vi "createMissionWaypoints.vi"(8 "error in (no error)":errorcluster, 11 "PassBuoys in":refnum<class "PassBuoys.lvclass">) -> (0 "error out":errorcluster, 3 "PassBuoys out":refnum<class "PassBuoys.lvclass">)   [LabVIEW 2011, in "PassBuoys.lvclass"]
doc: "Creates three waypoint objects for the mission, and puts them in the queue. The first waypoint is in front of the two buoys. The second is at their midpoint. The third is just past them."
uses:
  PassBuoys.lvclass
  PassBuoys.lvclass/PassBuoys.ctl
  2 Globals/2 Global.vi
  Waypoint/Waypoint.lvclass
panel:
  in  "Tolerance (meters)":dbl=3.0
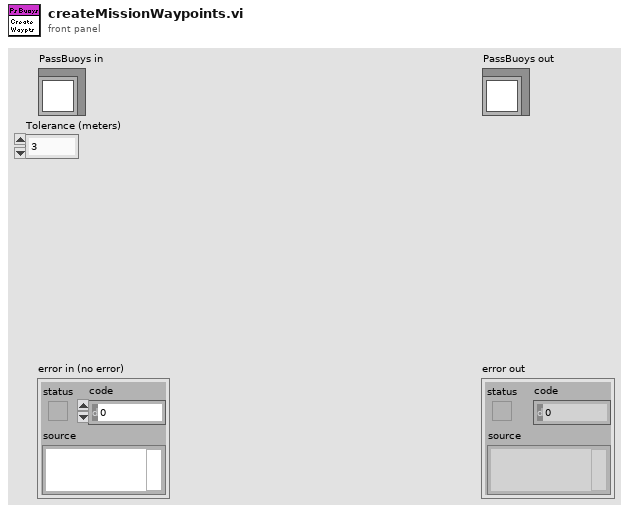
[diagram p1: front panel]
types:
  T1 = typedef "UTM Location.ctl" = cluster{"UTM Zone":dbl, "Hemisphere":enum16{"North", "South"}, "East":dbl, "North":dbl}
  T2 = typedef "UTM Circle.ctl" = cluster{"UTM Zone":dbl, "Hemisphere":enum16{"North", "South"}, "East":dbl, "North":dbl, "Radius":dbl}
  T3 = typedef "Waypoints List.ctl" = refnum<class "Waypoint.lvclass">[]
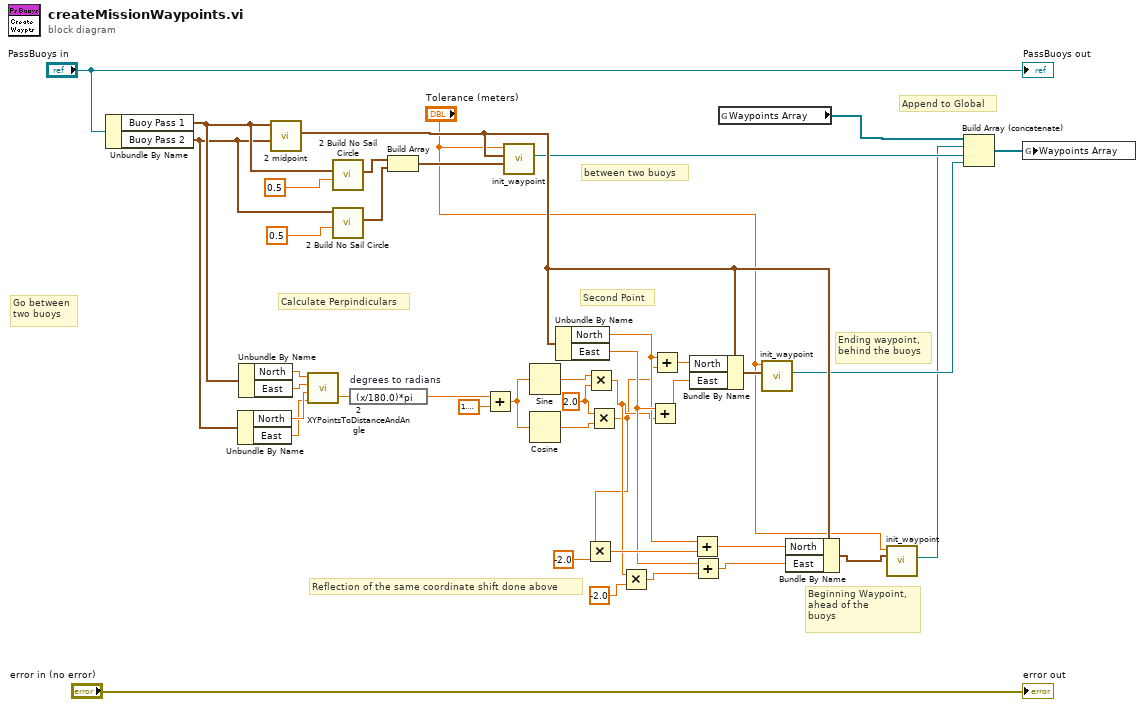
[diagram p0: block diagram]
diagram:
  w24 = 2.0 ("Tolerance (meters?)")
  # "Reflection of the same coordinate shift done above"
  # "between two buoys"
  # "Calculate Perpindiculars"
  # "Ending waypoint,\nbehind the buoys"
  # "Beginning Waypoint,\nahead of the\nbuoys"
  # "Second Point"
  # "Go between\ntwo buoys"
  # "Append to Global"
  n1 = Unbundle By Name("PassBuoys in") -> ("Buoy Pass 1"=w9:T1, "Buoy Pass 2"=w8:T1)
  n2 = Unbundle By Name(w8) -> ("North"=w32:dbl, "East"=w31:dbl)
  n3 = Unbundle By Name(w9) -> ("North"=w34:dbl, "East"=w33:dbl)
  n4 = call "2 midpoint.vi"("UTM 2"=w8, "UTM 1"=w9) -> ("Midpoint"=w15:T1)  [unwired: 8 in, 1 out]
  n5 = call "2 XYPointsToDistanceAndAngle.vi"("East 2"=w31, "North 2"=w32, "East 1"=w33, "North 1"=w34) -> ("Angle Diff"=w2:dbl)  [unwired: 1 out]
  n6 = call "2 Build No Sail Circle.vi"("Radius"=0.5, "UTM Location"=w9) -> ("UTM Circle"=w40:T2)  [unwired: 9 in]
  n7 = call "2 Build No Sail Circle.vi"("Radius"=0.5, "UTM Location"=w8) -> ("UTM Circle"=w38:T2)  [unwired: 9 in]
  n8 = expression code="(x/180.0)*pi" "degrees to radians"(w2) -> (w3:dbl)
  n9 = Build Array(w40, w38) -> (w41:T2[])
  n10 = Add(x=w3, y=1.5707963267948966) -> (x+y=w30:dbl)
  n11 = call "init_waypoint.vi"("No Sail Circles"=w41, "Coords"=w15, "Tolerance (m)"="Tolerance (meters)") -> ("Waypoint Out"=w12:refnum<class "Waypoint.lvclass">)  [unwired: 8 in]
  n12 = Sine(x=w30) -> (sin(x)=w26:dbl)
  n13 = Cosine(x=w30) -> (cos(x)=w25:dbl)
  n14 = Unbundle By Name(w15) -> ("North"=w18:dbl, "East"=w19:dbl)
  n15 = Multiply(x=w26, y=w24) -> (x*y=w6:dbl)
  n16 = Multiply(x=w24, y=w25) -> (x*y=w5:dbl)
  n17 = Multiply(x=w5, y=-2.0 ("Tolerance (meters?)")) -> (x*y=w20:dbl)
  n18 = Multiply(x=w6, y=-2.0 ("Tolerance (meters?)")) -> (x*y=w21:dbl)
  n19 = Add(x=w19, y=w6) -> (x+y=w29:dbl)
  n20 = Add(x=w18, y=w5) -> (x+y=w28:dbl)
  n21 = Bundle By Name(cluster=w15, "North"=w28, "East"=w29) -> (w27:T1)
  n22 = Add(x=w18, y=w20) -> (x+y=w17:dbl)
  n23 = Add(x=w19, y=w21) -> (x+y=w16:dbl)
  n24 = global read "2 Global.vi" "Waypoints Array"() -> (w36:T3)
  n25 = call "init_waypoint.vi"("Coords"=w27, "Tolerance (m)"="Tolerance (meters)") -> ("Waypoint Out"=w13:refnum<class "Waypoint.lvclass">)  [unwired: 9 in]
  n26 = Bundle By Name(cluster=w15, "North"=w17, "East"=w16) -> (w14:T1)
  n27 = call "init_waypoint.vi"("Coords"=w14, "Tolerance (m)"="Tolerance (meters)") -> ("Waypoint Out"=w11:refnum<class "Waypoint.lvclass">)  [unwired: 9 in]
  n28 = Build Array (concatenate)(w36, w11, w12, w13) -> (w35:T3)
  n29 = global write "2 Global.vi" "Waypoints Array"(w35) -> ()
  "error out" <- "error in (no error)"
  "PassBuoys out" <- "PassBuoys in"
